vi "Get Component Path.vi"(8 "Error In":errorcluster, 11 "Configuration":T1) -> (0 "Error Out":errorcluster, 2 "Component Install Paths":path[](array[path]), 3 "Configuration":T1)   [LabVIEW 2011, in "LVH-Build-Tools.lvlib"]
uses:
  LVH-Build-Tools.lvlib
  Type Defs/Configuration.ctl
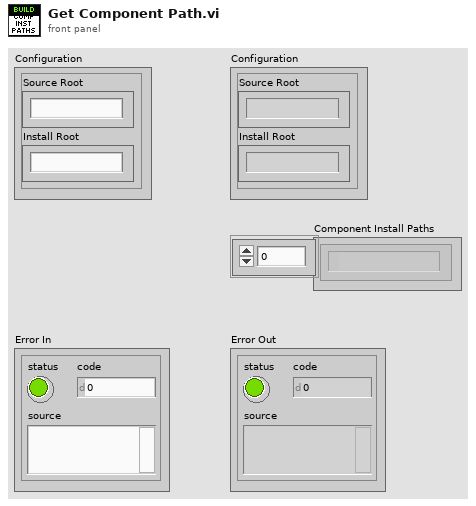
[diagram p1: front panel]
types:
  T1 = typedef "LVH-Build-Tools.lvlib/Configuration.ctl" = cluster{"Source Root":string, "Install Root":string, "Components":string[], "Ignore":string[]}
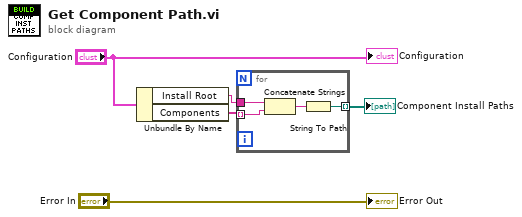
[diagram p0: block diagram]
diagram:
  n1 = Unbundle By Name("Configuration") -> ("Install Root"=w4:string, "Components"=w3:string[])
  n2 = for {
    tunnel: w4 -> [w9]
    tunnel: w3 -> [w8] mode=indexing
    tunnel: [w6] -> w1 mode=indexing
    n3 = Concatenate Strings(w9, w8) -> (w7:string)
    n4 = String To Path(string=w7) -> (path=w6:path)
  }
  "Component Install Paths" <- w1
  "Error Out" <- "Error In"
  "Configuration" <- "Configuration"
